vi "knownhosts_writeline.vi"() -> ()   [LabVIEW 2013]
doc: "Illustrates how to write host keys to a multi-line string."
uses:
  libssh2/libssh2_knownhost.ctl
  libssh2/Host Key Refnum.ctl
  libssh2/libssh2_init_default.vi
  libssh2/libssh2.lvlib
panel:
  out "error out":errorcluster
  out "output lines":string
  out "known hosts":T1[](array[typedef])
  in  "input lines":string="git.code.sf.net ssh-ed25519 AAAAC3NzaC1lZDI1NTE5AAAAIGObtXLh/mZom0pXjE5Mu211O+JvtzolqdNKVA+XJ466\ngit.code.sf.net ssh-rsa AAAAB3NzaC1yc2EAAAABIwAAAQEAoMesJ60dow5VqNsIqIQMBNmSYz6txSC5YSUXzPNWV4VIWTWdqbQoQuIu+oYGhBMoeaSWWCiVIDTwFDzQXrq8CwmyxWp+2TTuscKiOw830N2ycIVmm3ha0x6VpRGm37yo+z+bkQS3m/sE7bkfTU72GbeKufFHSv1VLnVy9nmJKFOraeKSHP/kjmatj9aC7Q2n8QzFWWjzMxVGg79TUs7sjm5KrtytbxfbLbKtrkn8OXsRy1ib9hKgOwg+"
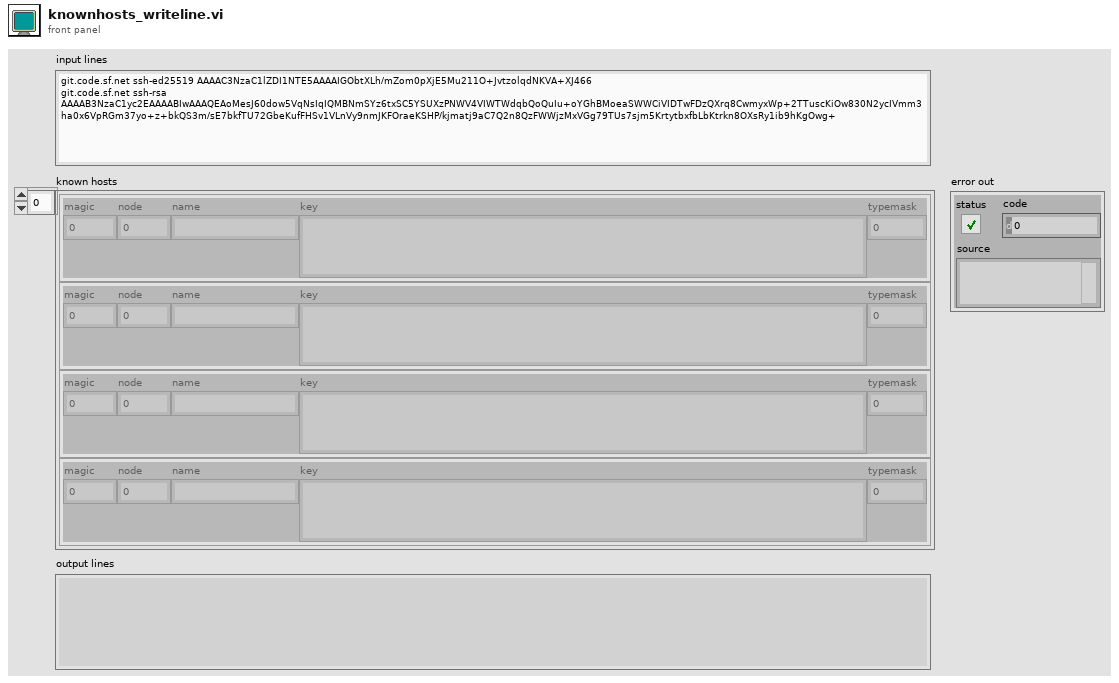
[diagram p1: front panel]
types:
  T1 = typedef "libssh2.lvlib/libssh2_knownhost.ctl" = cluster{"magic":u32, "node":u64, "name":string, "key":string, "typemask":i32}
  T2 = typedef "libssh2.lvlib/Host Key Refnum.ctl" = refnum<k1>
  T3 = typedef "libssh2.lvlib/Session Refnum.ctl" = refnum<k1>
  T4 = typedef "libssh2.lvlib/Host Key Database Refnum.ctl" = refnum<k1>
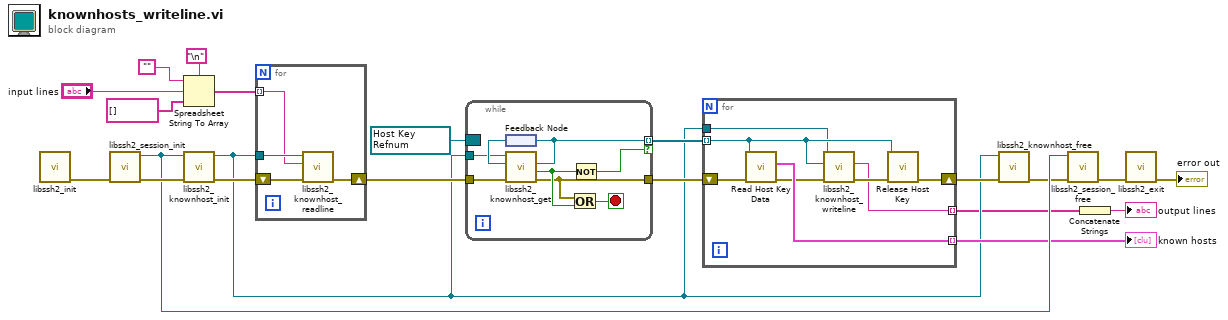
[diagram p0: block diagram]
diagram:
  w12 = T2 refnum items=["host key"] ("next")
  n1 = call-poly "libssh2_init.vi"() -> ("error out"=w21:errorcluster)  [unwired: 11 in]
  n2 = call "libssh2_session_init.vi"("error in (no error)"=w21) -> ("error out"=w20:errorcluster, "session"=w19:T3)  [unwired: 9 in]
  n3 = Spreadsheet String To Array(delimiter (Tab)="\n", format string="", spreadsheet string="input lines", array type (2D Dbl)=string[] []) -> (array=w9:string[])
  n4 = call "libssh2_knownhost_init.vi"("error in (no error)"=w20, "session"=w19) -> ("error out"=w16:errorcluster, "host key database"=w3:T4)  [unwired: 8 in]
  n5 = for {
    tunnel: w3 -> [w23]
    tunnel: w9 -> [w22] mode=indexing
    shift-right: [w24] -> w15
    shift-left: w16 -> [w25]
    n6 = call "libssh2_knownhost_readline.vi"("error in (no error)"=w25, "line"=w22, "host key database"=w23) -> ("error out"=w24:errorcluster)  [unwired: 8 in]
  }
  n7 = while {
    tunnel: w15 -> [w33]
    tunnel: [w26] -> w14
    tunnel: w3 -> [w30]
    border: w12 -> [_]
    tunnel: [w29] -> w11 mode=indexing if=w27
    stop <- w32 stop-if-true
    n8 = feedback #1() -> (w31:T2)
    n9 = call "libssh2_knownhost_get.vi"("error in (no error)"=w33, "previous host key"=w31, "host key database"=w30) -> ("error out"=w26:errorcluster, "end reached"=w28:bool, "host key"=w29:T2)  [unwired: 6 in]
    n10 = feedback-in #1(w29) -> ()
    n11 = Or(x=w26, y=w28) -> (x .or. y?=w32:bool)
    n12 = Not(x=w28) -> (.not. x?=w27:bool)
  }
  n13 = for {
    shift-right: [w41] -> w13
    shift-left: w14 -> [w40]
    tunnel: w11 -> [w36] mode=indexing
    tunnel: [w39] -> w4 mode=indexing
    tunnel: w3 -> [w35]
    tunnel: [w34] -> w2 mode=indexing
    n14 = call "Read Host Key Data.vi"("error in (no error)"=w40, "host key"=w36) -> ("error out"=w38:errorcluster, "host key data"=w39:T1)  [unwired: 8 in]
    n15 = call "libssh2_knownhost_writeline.vi"("error in (no error)"=w38, "host key"=w36, "host key database"=w35) -> ("error out"=w37:errorcluster, "line"=w34:string)  [unwired: 7 in]
    n16 = call "Release Host Key.vi"("error in (no error)"=w37, "host key"=w36) -> ("error out"=w41:errorcluster)  [unwired: 9 in]
  }
  "known hosts" <- w4
  n17 = call "libssh2_knownhost_free.vi"("error in (no error)"=w13, "host key database"=w3) -> ("error out"=w18:errorcluster)  [unwired: 9 in]
  n18 = call "libssh2_session_free.vi"("error in (no error)"=w18, "session"=w19) -> ("error out"=w17:errorcluster)  [unwired: 9 in]
  n19 = Concatenate Strings(w2) -> (→"output lines":string)
  n20 = call "libssh2_exit.vi"("error in (no error)"=w17) -> ("error out"=→"error out":errorcluster)  [unwired: 10 in]
